vi "Mouse State base FGV .vi"(7 "Method":enum16{"Get", "Set"}(ring), 8 "Error In":errorcluster, 11 "Mouse State In":T1) -> (0 "Error Out":errorcluster, 3 "Mouse State Out":T1)   [LabVIEW 2014]
uses:
  Controls/GMap Mouse States.ctl
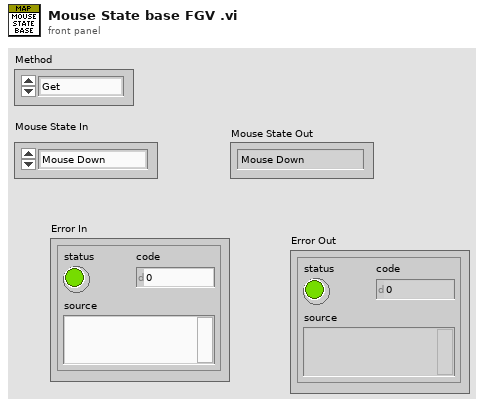
[diagram p1: front panel]
types:
  T1 = typedef "GMap Mouse States.ctl" = enum16{"Mouse Down", "Mouse Up"}
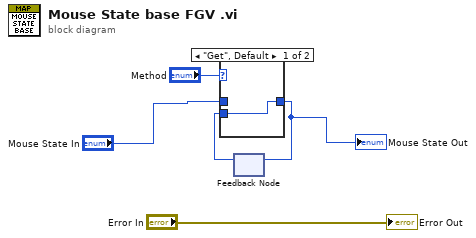
[diagram p0: block diagram]
diagram:
  n1 = feedback #1() -> (w4:T1)  [unwired: 1 in]
  n2 = case shown="\"Get\", Default" "Method" {
    tunnel: "Mouse State In" -> [_ w7]
    tunnel: [w6 w7] -> w3
    tunnel: w4 -> [w6 _]
    frame "Get", Default {
    }
    frame "Set" {
    }
  }
  "Mouse State Out" <- w3
  n3 = feedback-in #1(w3) -> ()
  "Error Out" <- "Error In"
